vi "3DIO.vi"(5 "DIO3 Refnum":refnum<k21>, 7 "DIO1 Refnum":refnum<k21>, 8 "DIR 3:0":fxp<+,4,4> format="%04b", 9 "OUT 3:0":fxp<+,4,4> format="%04b", 11 "DIO0 Refnum":refnum<k21>) -> (2 "IN 3:0":fxp<+,4,4> format="%04b")   [LabVIEW 2013]
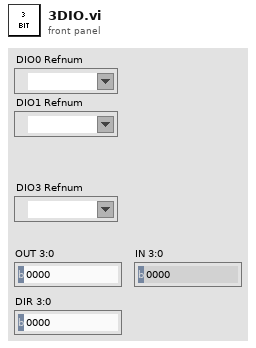
[diagram p1: front panel]
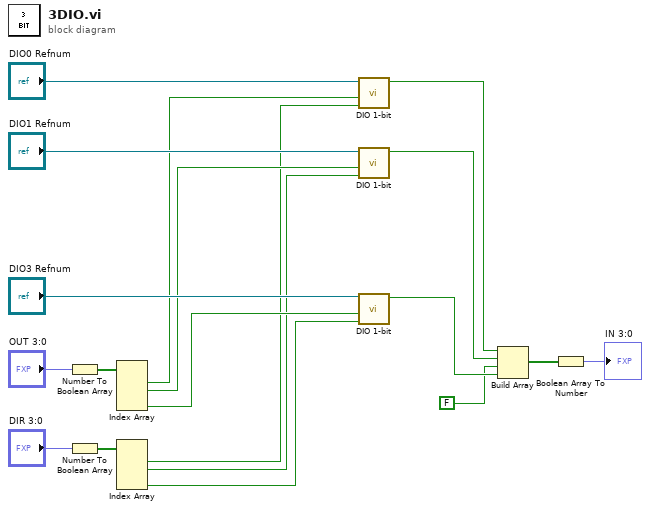
[diagram p0: block diagram]
diagram:
  n1 = Number To Boolean Array(number="OUT 3:0") -> (Boolean array=w14:bool[])
  n2 = Number To Boolean Array(number="DIR 3:0") -> (Boolean array=w10:bool[])
  n3 = Index Array(array=w14) -> (element #1=w13:bool, element #2=w12:bool, element #4=w11:bool)  [unwired: 4 in, 1 out]
  n4 = Index Array(array=w10) -> (element #1=w9:bool, element #2=w8:bool, element #4=w7:bool)  [unwired: 4 in, 1 out]
  n5 = call "DIO 1-bit.vi"("DIR"=w9, "OUT"=w13, "DIO Refnum"="DIO0 Refnum") -> ("IN"=w6:bool)  [unwired: 8 in]
  n6 = call "DIO 1-bit.vi"("DIR"=w8, "OUT"=w12, "DIO Refnum"="DIO1 Refnum") -> ("IN"=w5:bool)  [unwired: 8 in]
  n7 = call "DIO 1-bit.vi"("DIR"=w7, "OUT"=w11, "DIO Refnum"="DIO3 Refnum") -> ("IN"=w4:bool)  [unwired: 8 in]
  n8 = Build Array(w6, w5, FALSE ("element"), w4) -> (w3:bool[])
  n9 = Boolean Array To Number(Boolean array=w3) -> (number=→"IN 3:0":fxp<+,4,4>)
